vi "destroyEvnts.vi"(8 "error in (no error)":errorcluster, 11 "Electrometer in":refnum<class "Electrometer.lvclass">) -> (0 "error out":errorcluster, 3 "Electrometer out":refnum<class "Electrometer.lvclass">)   [LabVIEW 2016, in "Electrometer.lvclass"]
uses:
  Electrometer.lvclass
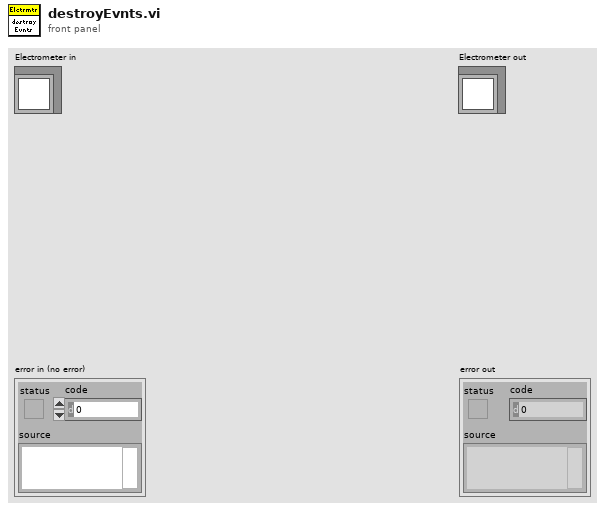
[diagram p1: front panel]
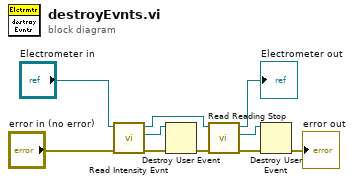
[diagram p0: block diagram]
diagram:
  n1 = call-dynamic "Read Intensity Evnt.vi"("error in (no error)"="error in (no error)", "Electrometer in"="Electrometer in") -> ("error out"=w7:errorcluster, "Intensity"=w8:refnum<user-event>, "Electrometer out"=w9:refnum<class "Electrometer.lvclass">)  [unwired: 7 in]
  n2 = Destroy User Event(user event=w8, error in=w7) -> (error out=w6:errorcluster)
  n3 = call-dynamic "Read Reading Stop.vi"("error in (no error)"=w6, "Electrometer in"=w9) -> ("error out"=w4:errorcluster, "ReadingStop"=w5:refnum<user-event>, "Electrometer out"=→"Electrometer out":refnum<class "Electrometer.lvclass">)  [unwired: 7 in]
  n4 = Destroy User Event(user event=w5, error in=w4) -> (error out=→"error out":errorcluster)
